vi "Auto Wait for Arm.vi"(11 "Run?":bool) -> (3 "Done":bool)   [LabVIEW 2013]
uses:
  Globals/Auto.vi
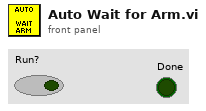
[diagram p1: front panel]
types:
  T1 = typedef "WPI_AnalogChannelDevRef.ctl" = cluster{"DevStatus":errorcluster, "Analog Module":T2, "Analog Channel":T3}
  T2 = typedef "FPGA_TypedefAnalogModule.ctl" = enum16{"Analog Module 1", "Analog Module 2"}
  T3 = typedef "FPGA_AIChannel.ctl" = enum8{"AI 1", "AI 2", "AI 3", "AI 4", "AI 5", "AI 6", "AI 7", "AI 8", "Invalid"}
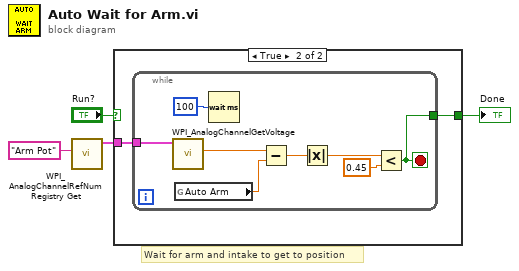
[diagram p0: block diagram]
diagram:
  # "Wait for arm and intake to get to position"
  n1 = call <vilib>:"WPI_AnalogChannelRefNum Registry Get.vi"("refnum name"="Arm Pot") -> ("AIDeviceRef"=w1:T1)  [unwired: 9 in, 1 out]
  n2 = case shown="True" "Run?" {
    selector: "Run?" -> [w5 _]
    tunnel: [w5 w6] -> w3
    tunnel: w1 -> [_ w7]
    frame False {
    }
    frame True {
      n3 = while {
        tunnel: w7 -> [w15]
        tunnel: [w8] -> w6
        stop <- w8 stop-if-true
        n4 = call <vilib>:"WPI_AnalogChannelGetVoltage.vi"("AIDeviceRef"=w15) -> ("Voltage"=w14:dbl)  [unwired: 8 in, 2 out]
        n5 = global read "Auto.vi" "Auto Arm"() -> (w13:dbl)
        n6 = Wait (ms)(milliseconds to wait=u32 100) -> ()  [unwired: 1 out]
        n7 = Subtract(x=w14, y=w13) -> (x-y=w12:dbl)
        n8 = Absolute Value(x=w12) -> (abs(x)=w11:dbl)
        n9 = Less?(x=w11, y=0.45) -> (x < y?=w8:bool)
      }
    }
  }
  "Done" <- w3
